vi "Single SSC DCPower Configure Single Point Force DC Current Symmetric Limits.vi"(0 "DCPower SSC in":T1, 1 "Current Level Range (A)":dbl format="%#_6p", 2 "Voltage Limit Range (V)":dbl format="%#_6p", 5 "Current Level (A)":dbl format="%#_6p", 7 "Voltage Limit (V)":dbl format="%#_6p", 11 "error in":errorcluster) -> (4 "DCPower SSC out":T1, 15 "error out":errorcluster)   [LabVIEW 2020]
doc: "This VI configures the sessions to force a single point DC current level with a voltage limit."
uses:
  SSC DCPower.ctl
  <instrlib>/niDCPower/nidcpower.llb/niDCPower Source Mode.ctl
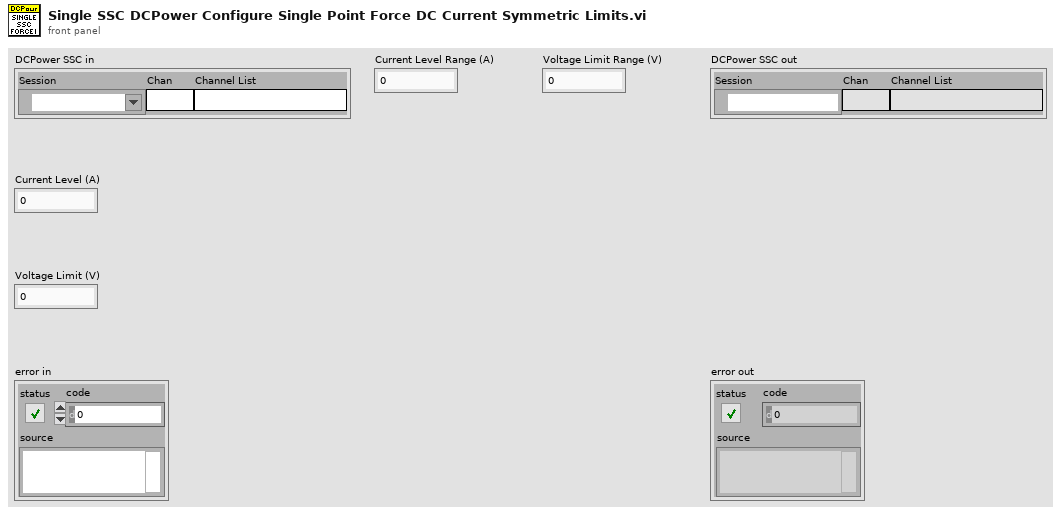
[diagram p1: front panel]
types:
  T1 = typedef "SSC DCPower.ctl" = cluster{"Session":refnum<k15>, "Chan":string, "Channel List":string}
  T2 = typedef "niDCPower Source Mode.ctl" = i32
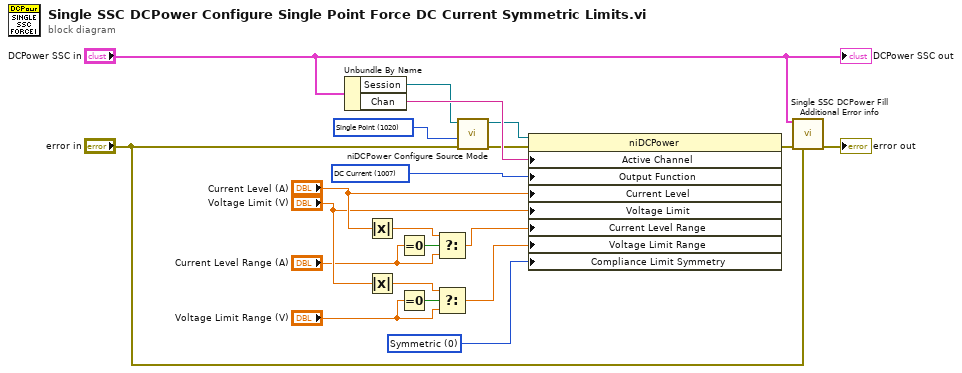
[diagram p0: block diagram]
diagram:
  w1 = 0 items=["Symmetric", "Asymmetric"] ("Source:Advanced:Compliance Limit Symmetry")
  w5 = T2 1020 items=["Single Point"=1020, "Sequence"=1021] ("source mode")
  w9 = 1007 items=["DC Voltage"=1006, "DC Current"=1007, "Pulse Voltage"=1049, "Pulse Current"=1050] ("Source:Output Function")
  n1 = Unbundle By Name("DCPower SSC in") -> ("Session"=w7:refnum<k15>, "Chan"=w10:string)
  n2 = Absolute Value(x="Current Level (A)") -> (abs(x)=w21:dbl)
  n3 = Absolute Value(x="Voltage Limit (V)") -> (abs(x)=w18:dbl)
  n4 = Equal To 0?(x="Current Level Range (A)") -> (x = 0?=w20:bool)
  n5 = Equal To 0?(x="Voltage Limit Range (V)") -> (x = 0?=w19:bool)
  n6 = Select(t=w21, s=w20, f="Current Level Range (A)") -> (s? t:f=w17:dbl)
  n7 = Select(t=w18, s=w19, f="Voltage Limit Range (V)") -> (s? t:f=w16:dbl)
  n8 = call <instrlib>:"niDCPower Configure Source Mode.vi"("error in (no error)"="error in", "source mode"=w5, "instrument handle"=w7) -> ("error out"=w8:errorcluster, "instrument handle out"=w6:refnum<k15>)  [unwired: 7 in]
  n9 = property class="niDCPower"(reference=w6, error in=w8, "Active Channel"=w10, "Output Function"=w9, "Current Level"="Current Level (A)", "Voltage Limit"="Voltage Limit (V)", "Current Level Range"=w17, "Voltage Limit Range"=w16, "Compliance Limit Symmetry"=w1) -> (error out=w15:errorcluster)  [unwired: 1 out]
  n10 = call "Single SSC DCPower Fill Additional Error info.vi"("DCPower SSC in"="DCPower SSC in", "error in"=w15, "previous error in"="error in") -> ("error out"=→"error out":errorcluster)  [unwired: 12 in]
  "DCPower SSC out" <- "DCPower SSC in"
